vi "ConfigEditor.vi"(11 "ConfigFile":path) -> ()   [LabVIEW 2012]
uses:
  Libs/Ini/ProcessMode.ctl
  Fun/Http/HttpClient.lvclass
  <vilib>/Utility/config.llb/Read Key (String).vi
  <vilib>/Utility/config.llb/Write Key (U32).vi
  <vilib>/Utility/config.llb/Write Key (String).vi
  Libs/Ini/IniReader&WriterForControl.lvlib
  <vilib>/Utility/config.llb/NI_LVConfig.lvlib
panel:
  in  "确定按钮":bool
  out "AllModelSetting":u32[](array[numeric])
  in  "Floor":string
  in  "Factory":string
  in  "选项卡控件":enum32{"Parameter", "DevList"}(tab)
  in  "FactoryStr":u16(ring) items=["五廠", "六廠"]
  in  "FloorStr":u16(ring) items=["一樓", "二樓", "三樓", "四樓"]
  out "FactoryCode":string
  out "FloorCode":string
  in  "Line":string
  in  "Port":refnum<visa-resource-name>
  in  "BaudRate":i32
  in  "LampBaudRate":i32
  in  "SerialRetry":i32
  in  "ReadDelay":i32
  in  "VerifyTimes":i32
  in  "DataUpload":bool
  in  "DataUrl":string
  in  "Delete":bool
  in  "Model":string(combo)
  in  "所有工位":cluster{"地址":string, "工位":string, "啟用":bool}[](array[cluster])
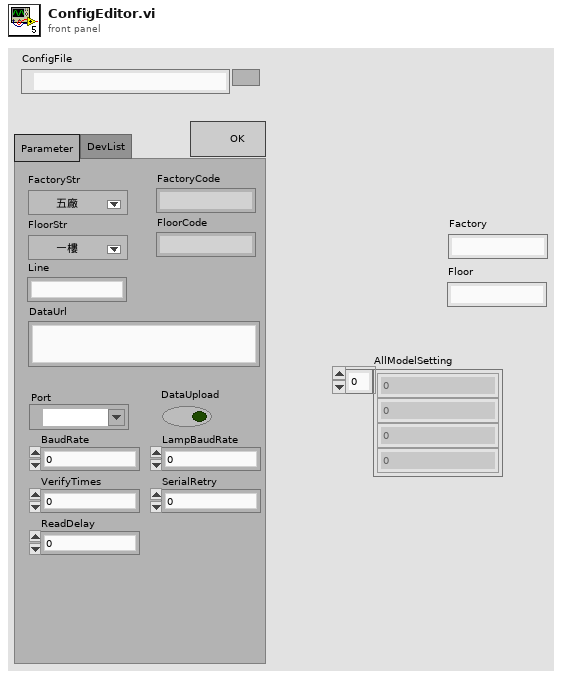
[diagram p1: front panel]
types:
  T1 = typedef "IniReader&WriterForControl.lvlib/ProcessMode.ctl" = enum16{"读", "写"}
  T2 = typedef "NI_LVConfig.lvlib/Config Data RefNum.ctl" = refnum<k1>
  T3 = cluster{"String":string, "trimmed string":string, bool}
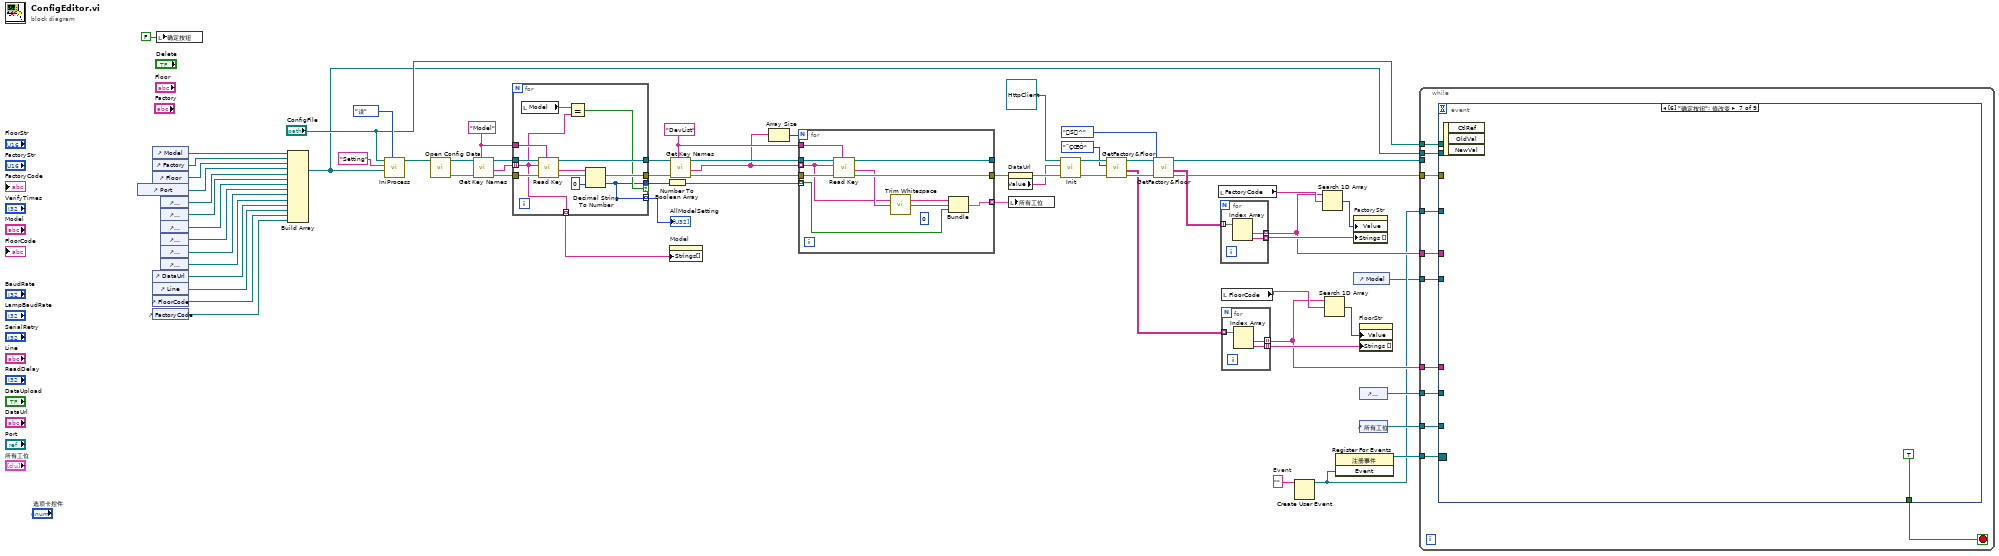
[diagram p0: block diagram]
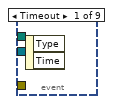
[diagram p2: hidden frame]
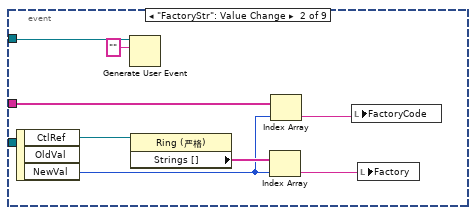
[diagram p3: hidden frame]
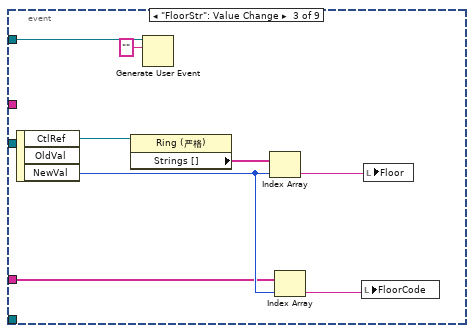
[diagram p4: hidden frame]
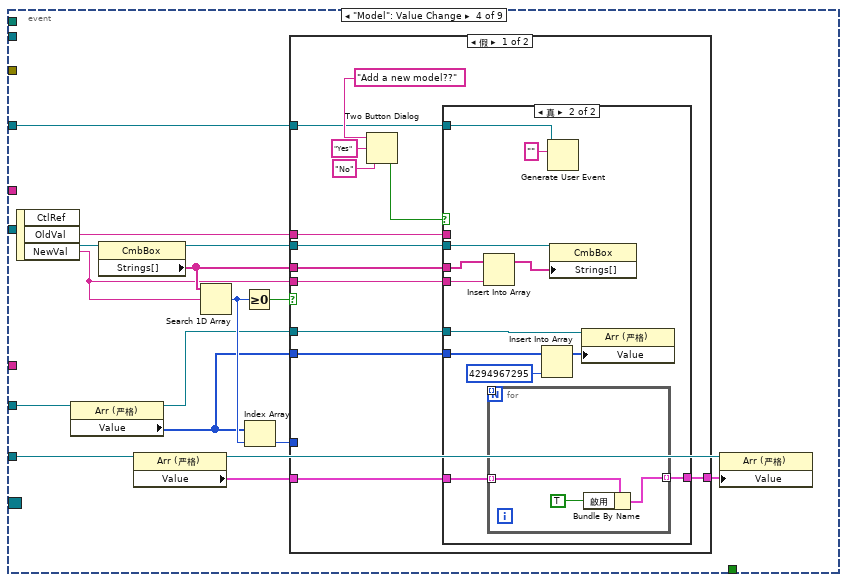
[diagram p5: hidden frame]
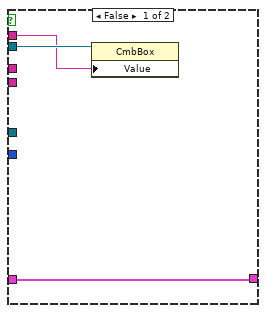
[diagram p6: hidden frame]
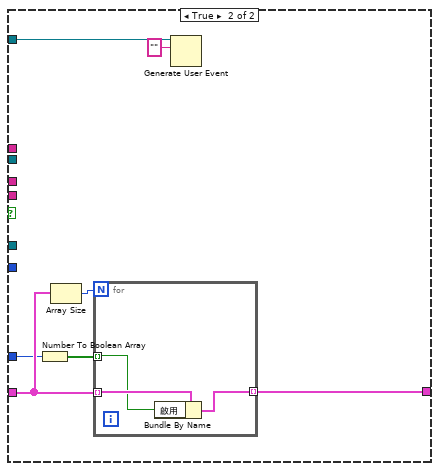
[diagram p7: hidden frame]
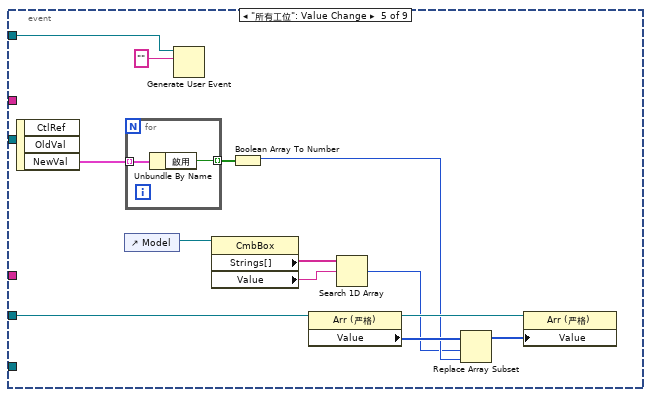
[diagram p8: hidden frame]
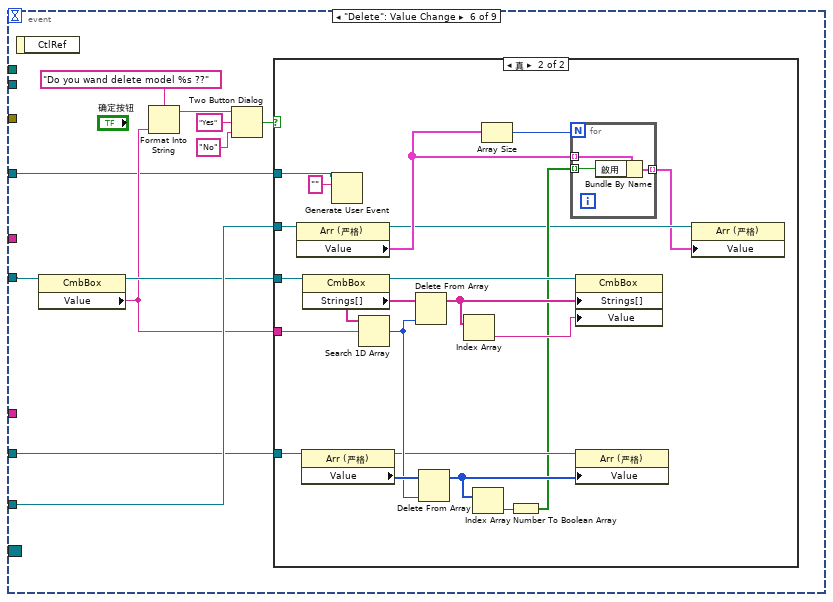
[diagram p9: hidden frame]
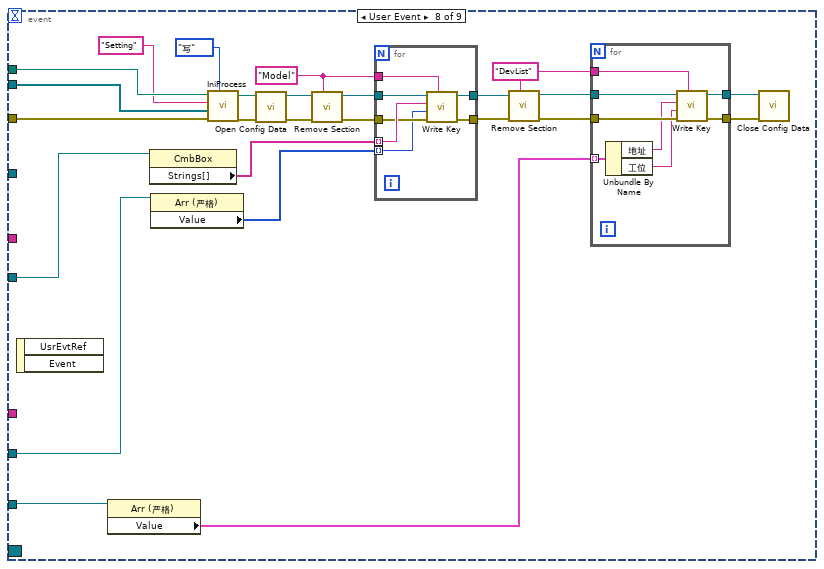
[diagram p11: hidden frame]
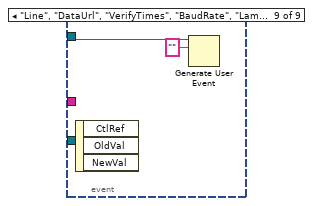
[diagram p12: hidden frame]
diagram:
  w6 = ""  # Event
  w39 = "DevList"
  w44 = "Model"
  n1 = control-ref of="Port"() -> (w63:refnum<vi>)
  n2 = control-ref of="Model"() -> (w66:refnum<vi>)
  n3 = control-ref of="Factory"() -> (w65:refnum<vi>)
  n4 = control-ref of="Floor"() -> (w64:refnum<vi>)
  n5 = control-ref of="DataUrl"() -> (w57:refnum<vi>)
  n6 = control-ref of="Line"() -> (w56:refnum<vi>)
  n7 = control-ref of="FloorCode"() -> (w55:refnum<vi>)
  n8 = control-ref of="FactoryCode"() -> (w54:refnum<vi>)
  n9 = local write "确定按钮"(FALSE ("确定按钮")) -> ()
  n10 = control-ref of="DataUpload"() -> (w53:refnum<vi>)
  n11 = control-ref of="ReadDelay"() -> (w62:refnum<vi>)
  n12 = control-ref of="SerialRetry"() -> (w61:refnum<vi>)
  n13 = control-ref of="LampBaudRate"() -> (w60:refnum<vi>)
  n14 = control-ref of="BaudRate"() -> (w59:refnum<vi>)
  n15 = control-ref of="VerifyTimes"() -> (w58:refnum<vi>)
  n16 = Build Array(w66, w65, w64, w63, w53, w62, w61, w60, w59, w58, w57, w56, w55, w54) -> (w3:refnum<vi>[])
  n17 = call "IniProcess.vi"("操作模式"=ProcessMode."读", "Ctls"=w3, "section"="Setting", "configuration file path"="ConfigFile") -> ("配置文件"=w50:path)  [unwired: 6 in, 1 out]
  n18 = call <vilib>:"Open Config Data.vi"("configuration file path"=w50) -> ("error out"=w48:errorcluster, "refnum"=w49:T2)  [unwired: 8 in, 1 out]
  n19 = call <vilib>:"Get Key Names.vi"("section"=w44, "error in (no error)"=w48, "refnum"=w49) -> ("error out"=w46:errorcluster, "key names"=w45:string[], "refnum out"=w47:T2)  [unwired: 5 in, 1 out]
  n20 = for {
    tunnel: w47 -> [w76]
    tunnel: w46 -> [w77]
    tunnel: w45 -> [w69] mode=indexing
    tunnel: [w75] -> w41
    tunnel: [w74] -> w40
    tunnel: w44 -> [w73]
    tunnel: [w69] -> w38 mode=indexing
    tunnel: [w67] -> w37 if=w68
    tunnel: [w67] -> w10 mode=indexing
    n21 = local read "Model"() -> (w70:string)
    n22 = call-poly <vilib>:"Read Key.vi"("section"=w73, "error in (no error)"=w77, "key"=w69, "refnum"=w76) -> ("error out"=w74:errorcluster, "value"=w72:string, "refnum out"=w75:T2)  [unwired: 4 in, 1 out]
    n23 = Equal?(x=w70, y=w69) -> (x = y?=w68:bool)
    n24 = Decimal String To Number(string=w72, default (0L)=u32 0) -> (number=w67:u32)  [unwired: 1 in, 1 out]
  }
  "AllModelSetting" <- w10
  n25 = Number To Boolean Array(number=w37) -> (Boolean array=w36:bool[])
  n26 = property on="Model" class="CmbBox"("Strings[]"=w38) -> ()  [unwired: 2 in, 2 out]
  n27 = call <vilib>:"Get Key Names.vi"("section"=w39, "error in (no error)"=w40, "refnum"=w41) -> ("error out"=w43:errorcluster, "key names"=w34:string[], "refnum out"=w42:T2)  [unwired: 5 in, 1 out]
  n28 = Array Size(array=w34) -> (size(s)=w35:i32)
  n29 = for {
    N: w35 -> [_]
    tunnel: w42 -> [w86]
    tunnel: w43 -> [w87]
    tunnel: w34 -> [w78] mode=indexing
    tunnel: [w85] -> _
    tunnel: [w84] -> w31
    tunnel: w39 -> [w83]
    tunnel: [w82] -> w33 mode=indexing
    tunnel: w36 -> [w80] mode=indexing
    (unwired) u8 0
    n30 = call-poly <vilib>:"Read Key.vi"("section"=w83, "error in (no error)"=w87, "key"=w78, "refnum"=w86) -> ("error out"=w84:errorcluster, "value"=w79:string, "refnum out"=w85:T2)  [unwired: 4 in, 1 out]
    n31 = call <vilib>:"Trim Whitespace.vi"("string"=w79) -> ("trimmed string"=w81:string)  [unwired: 1 in]
    n32 = Bundle("String"=w78, "trimmed string"=w81, w80) -> (w82:T3)  [unwired: 1 in]
  }
  n33 = property on="DataUrl" class="Str"(error in=w31) -> (error out=w30:errorcluster, "Value"=w29:string)  [unwired: 1 in, 1 out]
  n34 = local write "所有工位"(w33) -> ()
  n35 = call-dynamic "Init.vi"("error in (no error)"=w30, "Url"=w29, "HttpClient 输入"=refnum<class "HttpClient.lvclass"> refnum) -> ("error out"=w28:errorcluster, "HttpClient 输出"=w27:refnum<class "HttpClient.lvclass">)  [unwired: 7 in]
  n36 = call-dynamic "GetFactory&Floor.vi"("error in (no error)"=w28, "模式"=enum16{"˜ÇŒÓ", "S^"}."˜ÇŒÓ", "HttpClient 输入"=w27) -> ("error out"=w25:errorcluster, "Data"=w21:string[][], "HttpClient 输出"=w24:refnum<class "HttpClient.lvclass">)  [unwired: 6 in]
  n37 = call-dynamic "GetFactory&Floor.vi"("error in (no error)"=w25, "模式"=enum16{"˜ÇŒÓ", "S^"}."S^", "HttpClient 输入"=w24) -> ("error out"=w14:errorcluster, "Data"=w22:string[][], "HttpClient 输出"=w15:refnum<class "HttpClient.lvclass">)  [unwired: 6 in]
  n38 = local read "FactoryCode"() -> (w20:string)
  n39 = for {
    tunnel: w22 -> [w90] mode=indexing
    tunnel: [w89] -> w13 mode=indexing
    tunnel: [w88] -> w16 mode=indexing
    n40 = Index Array(array=w90) -> (element #1=w89:string, element #2=w88:string)  [unwired: 2 in]
  }
  n41 = for {
    tunnel: w21 -> [w93] mode=indexing
    tunnel: [w92] -> w11 mode=indexing
    tunnel: [w91] -> w12 mode=indexing
    n42 = Index Array(array=w93) -> (element #1=w92:string, element #2=w91:string)  [unwired: 2 in]
  }
  n43 = local read "FloorCode"() -> (w19:string)
  n44 = Create User Event(user event datatype=w6) -> (user event=w5:refnum<user-event>)  [unwired: 1 in, 1 out]
  n45 = Search 1D Array(1D array=w13, element=w20) -> (index of element=w18:i32)  [unwired: 1 in]
  n46 = Search 1D Array(1D array=w11, element=w19) -> (index of element=w17:i32)  [unwired: 1 in]
  n47 = register-events(w5) -> (reference out=w7:refnum<event-registration>)  [unwired: 2 in, 1 out]
  n48 = property on="FactoryStr" class="Ring (严格)"("Value"=w18, "Strings []"=w16) -> ()  [unwired: 2 in, 2 out]
  n49 = control-ref of="Model"() -> (w2:refnum<vi>)
  n50 = property on="FloorStr" class="Ring (严格)"("Value"=w17, "Strings []"=w12) -> ()  [unwired: 2 in, 2 out]
  n51 = control-ref of="AllModelSetting"() -> (w9:refnum<vi>)
  n52 = control-ref of="所有工位"() -> (w8:refnum<vi>)
  n53 = while {
    tunnel: w15 -> [_]
    tunnel: w14 -> [w96]
    tunnel: w13 -> [w104]
    tunnel: w11 -> [w103]
    tunnel: w9 -> [w102]
    tunnel: w8 -> [w101]
    tunnel: w7 -> [w100]
    tunnel: w5 -> [w99]
    tunnel: "ConfigFile" -> [w98]
    tunnel: w3 -> [w97]
    tunnel: w2 -> [w95]
    stop <- w94 stop-if-true
    n54 = event shown="[6] \"确定按钮\": 值改变" {
      selector: w100 -> [_ _ _ _ _ _ _ _ _]
      dyn-events: _ -> [_ _ _ _ _ _ _ _ _]
      timeout: _ -> [_ _ _ _ _ _ _ _ _]
      tunnel: w104 -> [_ w109 _ _ _ _ _ _ _]
      tunnel: w103 -> [_ _ w115 _ _ _ _ _ _]
      tunnel: w102 -> [_ _ _ w135 w187 w197 _ w240 _]
      tunnel: w101 -> [_ _ _ w131 _ w199 _ w236 _]
      tunnel: w99 -> [_ w106 w113 w121 w190 w194 _ _ w269]
      tunnel: w98 -> [_ _ _ _ _ _ _ w253 _]
      tunnel: w97 -> [_ _ _ _ _ _ _ w252 _]
      tunnel: w96 -> [_ _ _ _ _ _ _ w249 _]
      tunnel: w95 -> [_ _ _ _ _ w204 _ w229 _]
      tunnel: [_ _ _ _ _ _ TRUE _ _] -> w94
      event Timeout {
        n55 = event-data() -> ()  [unwired: 1 in, 2 out]
      }
      event "FactoryStr": Value Change {
        n56 = event-data() -> ("CtlRef"=w112:refnum<vi>, "NewVal"=w107:u16)  [unwired: 1 in, 1 out]
        n57 = Generate User Event(user event=w106, event data cluster="" ("事件数据")) -> ()  [unwired: 1 in, 2 out]
        n58 = property class="Ring (严格)"(reference=w112) -> ("Strings []"=w111:string[])  [unwired: 1 in, 2 out]
        n59 = Index Array(array=w111, index=w107) -> (element=w110:string)
        n60 = Index Array(array=w109, index=w107) -> (element=w108:string)
        n61 = local write "FactoryCode"(w108) -> ()
        n62 = local write "Factory"(w110) -> ()
      }
      event "FloorStr": Value Change {
        n63 = event-data() -> ("CtlRef"=w120:refnum<vi>, "NewVal"=w116:u16)  [unwired: 1 in, 1 out]
        n64 = property class="Ring (严格)"(reference=w120) -> ("Strings []"=w119:string[])  [unwired: 1 in, 2 out]
        n65 = Generate User Event(user event=w113, event data cluster="" ("事件数据")) -> ()  [unwired: 1 in, 2 out]
        n66 = Index Array(array=w119, index=w116) -> (element=w118:string)
        n67 = Index Array(array=w115, index=w116) -> (element=w117:string)
        n68 = local write "FloorCode"(w117) -> ()
        n69 = local write "Floor"(w118) -> ()
      }
      event "Model": Value Change {
        n70 = event-data() -> ("CtlRef"=w136:refnum<vi>, "OldVal"=w122:string, "NewVal"=w123:string)  [unwired: 1 in]
        n71 = property class="Arr (严格)"(reference=w135) -> (reference out=w127:refnum<vi>, "Value"=w126:u32[])  [unwired: 1 in, 1 out]
        n72 = property class="CmbBox"(reference=w136) -> (reference out=w125:refnum<vi>, "Strings[]"=w124:string[])  [unwired: 1 in, 1 out]
        n73 = property class="Arr (严格)"(reference=w131) -> (reference out=w129:refnum<vi>, "Value"=w130:cluster{"地址":string, "工位":string, "啟用":bool}[])  [unwired: 1 in, 1 out]
        n74 = Search 1D Array(1D array=w124, element=w123) -> (index of element=w133:i32)  [unwired: 1 in]
        n75 = Greater Or Equal To 0?(x=w133) -> (x >= 0?=w134:bool)
        n76 = Index Array(array=w126, index=w133) -> (element=w132:u32)
        n77 = case shown="假" w134 {
          tunnel: w132 -> [_ w173]
          tunnel: w130 -> [w149 w174]
          tunnel: [w148 w171] -> w128
          tunnel: w127 -> [w144 _]
          tunnel: w126 -> [w143 _]
          tunnel: w125 -> [w145 _]
          tunnel: w124 -> [w147 _]
          tunnel: w123 -> [w146 _]
          tunnel: w122 -> [w138 _]
          tunnel: w121 -> [w137 w169]
          frame False {
            n78 = Two Button Dialog(message="Add a new model??", 1:"No" ("F按钮名称（“取消”）"), 2:"Yes" ("T按钮名称（“确定”）")) -> (T button?=w142:bool)
            n79 = case shown="真" w142 {
              tunnel: w149 -> [w152 w164]
              tunnel: [w152 w163] -> w148
              tunnel: w147 -> [_ w162]
              tunnel: w146 -> [_ w161]
              tunnel: w145 -> [w151 w160]
              tunnel: w144 -> [_ w158]
              tunnel: w143 -> [_ w157]
              tunnel: w138 -> [w150 _]
              tunnel: w137 -> [_ w153]
              frame False {
                n80 = property class="CmbBox"(reference=w151, "Value"=w150) -> ()  [unwired: 1 in, 2 out]
              }
              frame True {
                n81 = Insert Into Array(array=w162, new element=w161) -> (w159:string[])  [unwired: 1 in]
                n82 = for {
                  N -> [w165]
                  tunnel: w164 -> [w168] mode=indexing
                  tunnel: [w166] -> w163 mode=indexing
                  tunnel: [w165] -> _ mode=indexing
                  n83 = Bundle By Name(cluster=w168, "啟用"=TRUE) -> (w166:cluster{"地址":string, "工位":string, "啟用":bool})
                }
                n84 = Insert Into Array(array=w157, new element=u32 4294967295 ("新元素/子数组")) -> (w156:u32[])  [unwired: 1 in]
                n85 = Generate User Event(user event=w153, event data cluster="" ("事件数据")) -> ()  [unwired: 1 in, 2 out]
                n86 = property class="CmbBox"(reference=w160, "Strings[]"=w159) -> ()  [unwired: 1 in, 2 out]
                n87 = property class="Arr (严格)"(reference=w158, "Value"=w156) -> ()  [unwired: 1 in, 2 out]
              }
            }
          }
          frame True {
            n88 = Number To Boolean Array(number=w173) -> (Boolean array=w172:bool[])
            n89 = Array Size(array=w174) -> (size(s)=w175:i32)
            n90 = for {
              N: w175 -> [_]
              tunnel: w174 -> [w178] mode=indexing
              tunnel: w172 -> [w177] mode=indexing
              tunnel: [w176] -> w171 mode=indexing
              n91 = Bundle By Name(cluster=w178, "啟用"=w177) -> (w176:cluster{"地址":string, "工位":string, "啟用":bool})
            }
            n92 = Generate User Event(user event=w169, event data cluster="" ("事件数据")) -> ()  [unwired: 1 in, 2 out]
          }
        }
        n93 = property class="Arr (严格)"(reference=w129, "Value"=w128) -> ()  [unwired: 1 in, 2 out]
      }
      event "所有工位": Value Change {
        n94 = event-data() -> ("NewVal"=w189:cluster{"地址":string, "工位":string, "啟用":bool}[])  [unwired: 1 in, 2 out]
        n95 = control-ref of="Model"() -> (w186:refnum<vi>)
        n96 = for {
          tunnel: w189 -> [w193] mode=indexing
          tunnel: [w192] -> w188 mode=indexing
          n97 = Unbundle By Name(w193) -> ("啟用"=w192:bool)
        }
        n98 = Generate User Event(user event=w190, event data cluster="" ("事件数据")) -> ()  [unwired: 1 in, 2 out]
        n99 = property class="CmbBox"(reference=w186) -> ("Strings[]"=w185:string[], "Value"=w184:string)  [unwired: 1 in, 2 out]
        n100 = Boolean Array To Number(Boolean array=w188) -> (number=w181:u32)
        n101 = property class="Arr (严格)"(reference=w187) -> (reference out=w183:refnum<vi>, "Value"=w182:u32[])  [unwired: 1 in, 1 out]
        n102 = Search 1D Array(1D array=w185, element=w184) -> (index of element=w180:i32)  [unwired: 1 in]
        n103 = Replace Array Subset(array=w182, new element=w181, index=w180) -> (w179:u32[])
        n104 = property class="Arr (严格)"(reference=w183, "Value"=w179) -> ()  [unwired: 1 in, 2 out]
      }
      event "Delete": Value Change {
        n105 = event-data() -> ()  [unwired: 1 in, 1 out]
        n106 = property class="CmbBox"(reference=w204) -> (reference out=w196:refnum<vi>, "Value"=w195:string)  [unwired: 1 in, 1 out]
        n107 = Format Into String(format string="Do you wand delete model %s ??" ("格式字符串"), w195) -> (resulting string=w202:string)  [unwired: 2 in, 1 out]
        n108 = Two Button Dialog(message=w202, 1:"No" ("T按钮名称（“确定”）"), 2:"Yes" ("T按钮名称（“确定”）")) -> (T button?=w198:bool)
        n109 = case shown="真" w198 {
          tunnel: w199 -> [_ w224]
          tunnel: w197 -> [_ w219]
          tunnel: w196 -> [_ w223]
          tunnel: w195 -> [_ w222]
          tunnel: w194 -> [_ w205]
          frame False {
          }
          frame True {
            n110 = property class="Arr (严格)"(reference=w224) -> (reference out=w208:refnum<vi>, "Value"=w211:cluster{"地址":string, "工位":string, "啟用":bool}[])  [unwired: 1 in, 1 out]
            n111 = property class="Arr (严格)"(reference=w219) -> (reference out=w216:refnum<vi>, "Value"=w218:u32[])  [unwired: 1 in, 1 out]
            n112 = property class="CmbBox"(reference=w223) -> (reference out=w220:refnum<vi>, "Strings[]"=w221:string[])  [unwired: 1 in, 1 out]
            n113 = Generate User Event(user event=w205, event data cluster="" ("事件数据")) -> ()  [unwired: 1 in, 2 out]
            n114 = Search 1D Array(1D array=w221, element=w222) -> (index of element=w217:i32)  [unwired: 1 in]
            n115 = Delete From Array(array=w221, index=w217) -> (array with subset deleted=w215:string[])  [unwired: 1 in, 1 out]
            n116 = Delete From Array(array=w218, index=w217) -> (array with subset deleted=w213:u32[])  [unwired: 1 in, 1 out]
            n117 = Index Array(array=w215) -> (element=w214:string)  [unwired: 1 in]
            n118 = Index Array(array=w213) -> (element=w212:u32)  [unwired: 1 in]
            n119 = Array Size(array=w211) -> (size(s)=w210:i32)
            n120 = Number To Boolean Array(number=w212) -> (Boolean array=w209:bool[])
            n121 = for {
              N: w210 -> [_]
              tunnel: w211 -> [w227] mode=indexing
              tunnel: w209 -> [w226] mode=indexing
              tunnel: [w225] -> w207 mode=indexing
              n122 = Bundle By Name(cluster=w227, "啟用"=w226) -> (w225:cluster{"地址":string, "工位":string, "啟用":bool})
            }
            n123 = property class="CmbBox"(reference=w220, "Strings[]"=w215, "Value"=w214) -> ()  [unwired: 1 in, 2 out]
            n124 = property class="Arr (严格)"(reference=w216, "Value"=w213) -> ()  [unwired: 1 in, 2 out]
            n125 = property class="Arr (严格)"(reference=w208, "Value"=w207) -> ()  [unwired: 1 in, 2 out]
          }
        }
      }
      event "确定按钮": Value Change {
        n126 = event-data() -> ()  [unwired: 1 in, 3 out]
      }
      event User Event {
        w232 = "DevList" ("section")
        w242 = "Model" ("section")
        n127 = event-data() -> ()  [unwired: 1 in, 2 out]
        n128 = property class="Arr (严格)"(reference=w236) -> ("Value"=w235:cluster{"地址":string, "工位":string, "啟用":bool}[])  [unwired: 1 in, 2 out]
        n129 = property class="CmbBox"(reference=w229) -> ("Strings[]"=w241:string[])  [unwired: 1 in, 2 out]
        n130 = property class="Arr (严格)"(reference=w240) -> ("Value"=w239:u32[])  [unwired: 1 in, 2 out]
        n131 = call "IniProcess.vi"("操作模式"=ProcessMode."写", "error in (no error)"=w249, "Ctls"=w252, "section"="Setting", "configuration file path"=w253) -> ("error out"=w248:errorcluster, "配置文件"=w247:path)  [unwired: 5 in]
        n132 = call <vilib>:"Open Config Data.vi"("error in (no error)"=w248, "configuration file path"=w247) -> ("error out"=w246:errorcluster, "refnum"=w245:T2)  [unwired: 7 in, 1 out]
        n133 = call <vilib>:"Remove Section.vi"("section"=w242, "error in (no error)"=w246, "refnum"=w245) -> ("error out"=w244:errorcluster, "refnum out"=w243:T2)  [unwired: 6 in, 1 out]
        n134 = for {
          tunnel: w244 -> [w265]
          tunnel: w243 -> [w268]
          tunnel: w242 -> [w267]
          tunnel: w241 -> [w266] mode=indexing
          tunnel: w239 -> [w264] mode=indexing
          tunnel: [w263] -> w238
          tunnel: [w262] -> w237
          n135 = call-poly <vilib>:"Write Key.vi"("section"=w267, "error in (no error)"=w265, "value"=w264, "key"=w266, "refnum"=w268) -> ("error out"=w263:errorcluster, "refnum out"=w262:T2)  [unwired: 4 in, 1 out]
        }
        n136 = call <vilib>:"Remove Section.vi"("section"=w232, "error in (no error)"=w238, "refnum"=w237) -> ("error out"=w233:errorcluster, "refnum out"=w234:T2)  [unwired: 6 in, 1 out]
        n137 = for {
          tunnel: w235 -> [w261] mode=indexing
          tunnel: w234 -> [w259]
          tunnel: w233 -> [w260]
          tunnel: w232 -> [w256]
          tunnel: [w255] -> w231
          tunnel: [w254] -> w230
          n138 = Unbundle By Name(w261) -> ("地址"=w258:string, "工位"=w257:string)
          n139 = call-poly <vilib>:"Write Key.vi"("section"=w256, "error in (no error)"=w260, "value"=w257, "key"=w258, "refnum"=w259) -> ("error out"=w255:errorcluster, "refnum out"=w254:T2)  [unwired: 4 in, 1 out]
        }
        n140 = call <vilib>:"Close Config Data.vi"("error in (no error)"=w231, "refnum"=w230) -> ()  [unwired: 8 in, 2 out]
      }
      event "Line", "DataUrl", "VerifyTimes", "BaudRate", "LampBaudRate", "SerialRetry", "ReadDelay", "DataUpload", "Port": Value Change {
        n141 = event-data() -> ()  [unwired: 1 in, 3 out]
        n142 = Generate User Event(user event=w269, event data cluster="" ("事件数据")) -> ()  [unwired: 1 in, 2 out]
      }
    }
  }
